vi "IntakeNetworkSlow.vi"(8 "error in (no error)":errorcluster) -> (0 "error out":errorcluster)   [LabVIEW 2023]
uses:
  IntakeGlobal.vi
  <vilib>/Rock Robotics/Network Tables/NT Read Number.vi
  <vilib>/Rock Robotics/Network Tables/NT Write Number.vi
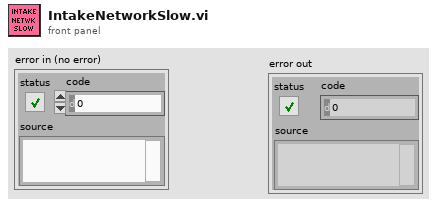
[diagram p1: front panel]
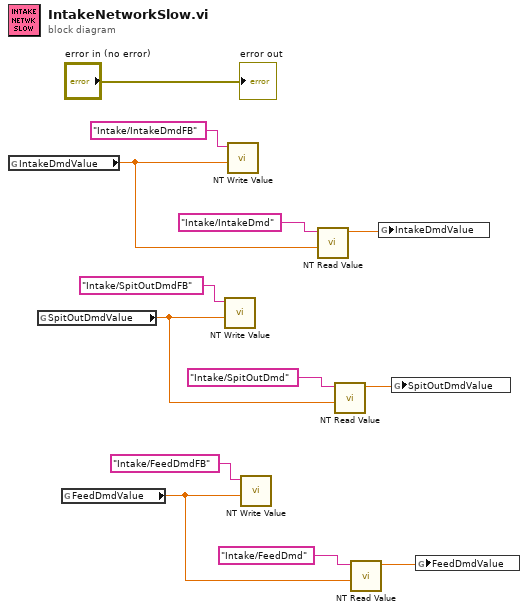
[diagram p0: block diagram]
diagram:
  n1 = global read "IntakeGlobal.vi" "IntakeDmdValue"() -> (w8:dbl)
  n2 = global read "IntakeGlobal.vi" "SpitOutDmdValue"() -> (w5:dbl)
  n3 = global read "IntakeGlobal.vi" "FeedDmdValue"() -> (w1:dbl)
  n4 = call-poly <vilib>:"NT Write Value.vi"("value"=w5, "name"="Intake/SpitOutDmdFB") -> ()  [unwired: 9 in, 1 out]
  n5 = call-poly <vilib>:"NT Write Value.vi"("value"=w8, "name"="Intake/IntakeDmdFB") -> ()  [unwired: 9 in, 1 out]
  n6 = call-poly <vilib>:"NT Write Value.vi"("value"=w1, "name"="Intake/FeedDmdFB") -> ()  [unwired: 9 in, 1 out]
  n7 = call-poly <vilib>:"NT Read Value.vi"("default value"=w8, "name"="Intake/IntakeDmd") -> ("value"=w9:dbl)  [unwired: 7 in, 2 out]
  n8 = call-poly <vilib>:"NT Read Value.vi"("default value"=w5, "name"="Intake/SpitOutDmd") -> ("value"=w6:dbl)  [unwired: 7 in, 2 out]
  n9 = call-poly <vilib>:"NT Read Value.vi"("default value"=w1, "name"="Intake/FeedDmd") -> ("value"=w2:dbl)  [unwired: 7 in, 2 out]
  n10 = global write "IntakeGlobal.vi" "IntakeDmdValue"(w9) -> ()
  n11 = global write "IntakeGlobal.vi" "SpitOutDmdValue"(w6) -> ()
  n12 = global write "IntakeGlobal.vi" "FeedDmdValue"(w2) -> ()
  "error out" <- "error in (no error)"
